vi "To Variant.vi"(0 "Obj in":refnum<class "State.lvclass">, 11 "error in (no error)":errorcluster) -> (4 "Obj out":refnum<class "State.lvclass">, 8 "Array":variant[](array[variant]), 15 "error out":errorcluster)   [LabVIEW 2020, in "State.lvclass"]
uses:
  State.lvclass
  State.lvclass/State.ctl
  epl-vi-lib/Koop/KObject Class/KObject.lvclass
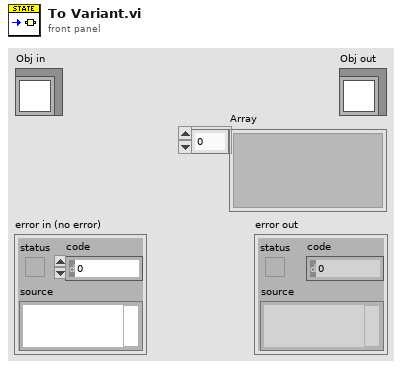
[diagram p1: front panel]
types:
  T1 = typedef "State.lvclass/Serialized.ctl" = cluster{"Name":string, "TTL-only":bool, "Timeouts":refnum<class "Timeout.lvclass">[], "Term":refnum<class "Termination.lvclass">[], "SigMan":refnum<class "SignalManager.lvclass">, "Grating":T2, "Execute script":bool}
  T2 = typedef "Tosca-Grating.ctl" = cluster{"Type":T3, "Orientation (deg)":dbl, "Spatial frequency (cpd)":dbl, "Velocity (Hz)":dbl, "Contrast":dbl, "Background intensity":dbl, "Duration (ms)":dbl, "Phase (cycles)":dbl}
  T3 = typedef "Tosca-Grating Type.ctl" = enum16{"OFF", "Square", "Sine"}
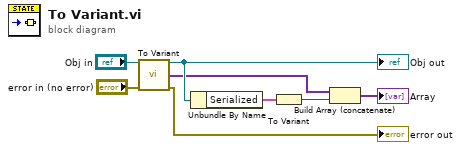
[diagram p0: block diagram]
diagram:
  n1 = call-parent "To Variant.vi"("KObject in"="Obj in", "error in (no error)"="error in (no error)") -> ("KObject out"=w3:refnum<class "State.lvclass">, "Array"=w2:variant[], "error out"=→"error out":errorcluster)  [unwired: 11 in]
  "Obj out" <- w3
  n2 = Unbundle By Name(w3) -> ("Serialized"=w4:T1)
  n3 = To Variant(anything=w4) -> (Variant=w5:variant)
  n4 = Build Array (concatenate)(w2, w5) -> (→"Array":variant[])
